vi "Initialize Lookup Table - Sin Syn.vi"() -> ()   [LabVIEW 2015]
uses:
  <vilib>/measure/NI_MABase.lvlib
panel:
  out "波形图":i16[](graph)
  out "Init Data Out":i16[](array[numeric])
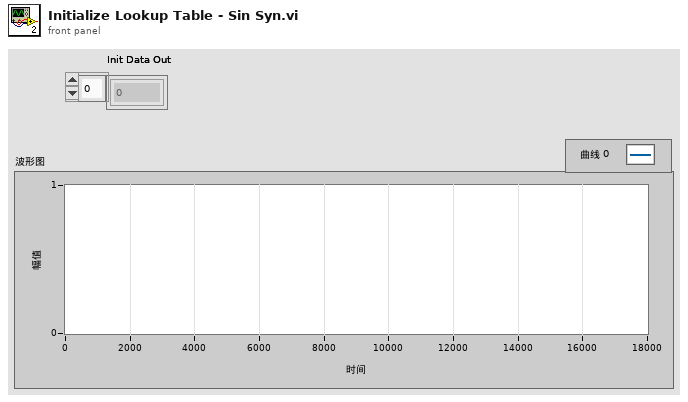
[diagram p1: front panel]
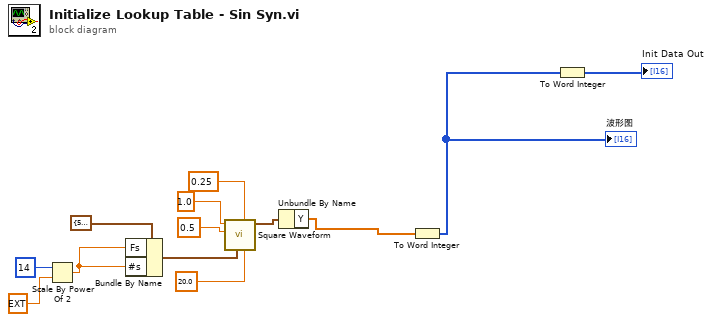
[diagram p0: block diagram]
diagram:
  n1 = Scale By Power Of 2(n=i16 14, x=ext 1.0) -> (x*2^n=w10:ext)
  n2 = Bundle By Name(cluster=cluster{"Fs":dbl, "#s":dbl} {"Fs"=5000.0, "#s"=50.0} ("sampling info"), "Fs"=w10, "#s"=w10) -> (w7:cluster{"Fs":dbl, "#s":dbl})
  n3 = call <vilib>:"Square Waveform.vi"("duty cycle (%)"=20.0, "offset"=0.25, "sampling info"=w7, "amplitude"=0.5, "frequency"=1.0) -> ("signal out"=w6:waveform(dbl))  [unwired: 5 in, 1 out]
  n4 = Unbundle By Name(w6) -> ("Y"=w3:dbl[])
  n5 = To Word Integer(number=w3) -> (16bit integer=w4:i16[])
  "波形图" <- w4
  n6 = To Word Integer(number=w4) -> (16bit integer=→"Init Data Out":i16[])
